vi "Fifo2File.vi"(8 "file refnum in":refnum<file>, 9 "FIFO size":u32, 11 "rf fifo Input":refnum<k33>) -> (0 "file refnum out":refnum<file>, 1 "fifo full counter":u16, 3 "rt fifo output":refnum<k33>)   [LabVIEW 2010, in "KevLib01.lvlib"]
uses:
  KevLib01.lvlib
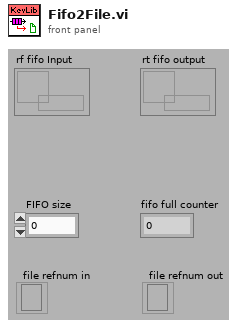
[diagram p1: front panel]
types:
  T1 = enum16{"big-endian, network order", "native, host order", "little-endian"}
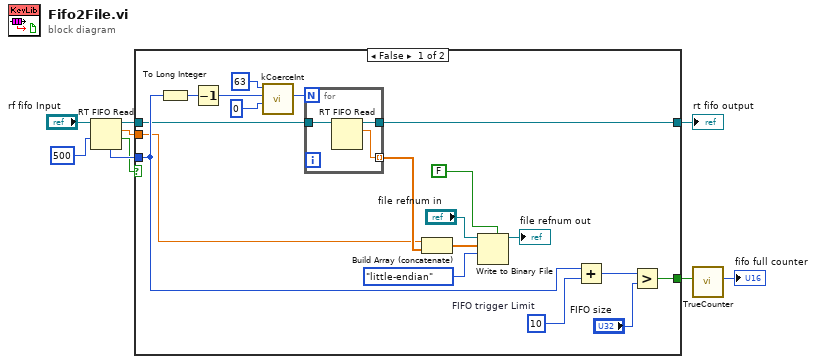
[diagram p0: block diagram]
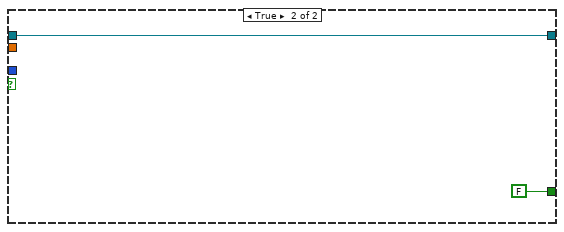
[diagram p2: hidden frame]
diagram:
  n1 = RT FIFO Read(0:"rf fifo Input", 2:500 ("timeout in ms (0)")) -> (7:w9:u32, 8:w6:refnum<k33>, 9:w8:dbl, 10:w3:bool)  [unwired: 2 in, 1 out]
  n2 = case shown="False" w3 {
    tunnel: [w28 FALSE] -> w2
    tunnel: w9 -> [w24 _]
    tunnel: w8 -> [w21 _]
    tunnel: [w20 w32] -> w7
    tunnel: w6 -> [w19 w32]
    frame False {
      w25 = u32 10  # FIFO trigger Limit
      n3 = To Long Integer(number=w24) -> (32bit integer=w14:i32)
      n4 = Decrement(x=w14) -> (x-1=w13:i32)
      n5 = call "kCoerceInt.vi"("lower"=0 ("lower limit"), "input"=w13, "upper"=63 ("upper limit")) -> ("output"=w10:i32)  [unwired: 8 out]
      n6 = for {
        N: w10 -> [_]
        tunnel: w19 -> [w31]
        tunnel: [w30] -> w20
        tunnel: [w29] -> w22 mode=indexing
        n7 = RT FIFO Read(0:w31) -> (8:w30:refnum<k33>, 9:w29:dbl)  [unwired: 2 in, 4 out]
      }
      n8 = Build Array (concatenate)(w21, w22) -> (w23:dbl[])
      n9 = Write to Binary File(file (use dialog)="file refnum in", data=w23, 5:FALSE ("prepend array or string size? (T)"), 9:T1."little-endian" ("byte order (0:big-endian, network order)")) -> (refnum out=→"file refnum out":refnum<file>)  [unwired: 1 in, 3 out]
      n10 = Add(x=w24, y=w25) -> (x+y=w27:u32)
      n11 = Greater?(x=w27, y="FIFO size") -> (0:w28:bool)
    }
    frame True {
    }
  }
  "rt fifo output" <- w7
  n12 = call "TrueCounter.vi"("True?"=w2) -> ("True Count"=→"fifo full counter":u16)  [unwired: 10 out]
